vi "Emballage_BDD_correspondance_Code_barre.vi"(7 "tableau des codes barres":string[](array[string]), 8 "entrée d'erreur (pas d'erreur)":errorcluster, 9 "tableau des produits code FAS":string[](array[string]), 10 "Etiquette scanné":string, 11 "MulticolumnListbox en entrée":refnum<vi>) -> (0 "sortie d'erreur":errorcluster, 1 "index_produit":i32, 2 "message":string, 3 "Produit Code FAS":string)   [LabVIEW 2020]
uses:
  Modules/FS/60_FS_Controles/60_FS_SetGet.ctl
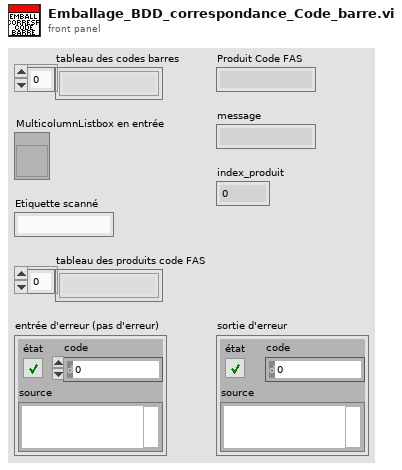
[diagram p1: front panel]
types:
  T1 = typedef "60_FS_SetGet.ctl" = enum16{"set", "get"}
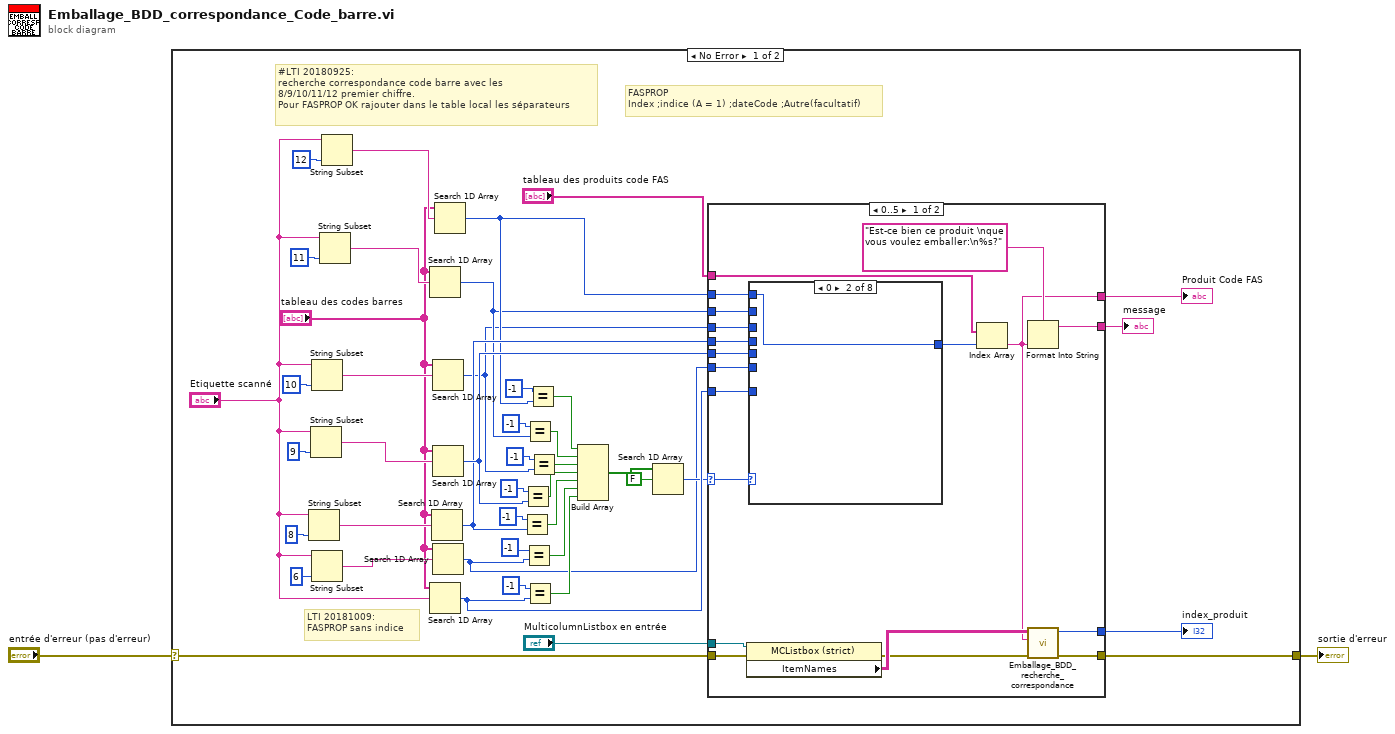
[diagram p0: block diagram]
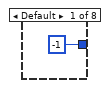
[diagram p2: hidden frame]
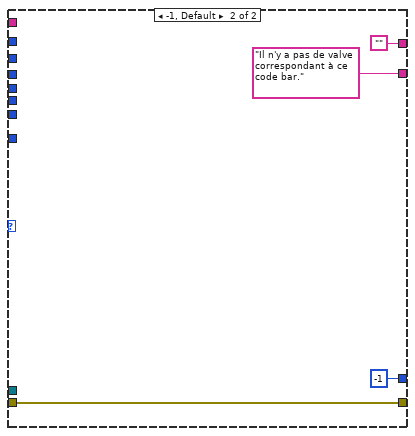
[diagram p9: hidden frame]
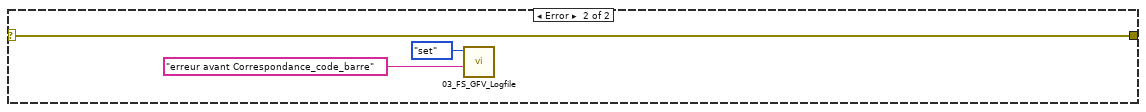
[diagram p10: hidden frame]
diagram:
  n1 = case shown="No Error" "entrée d'erreur (pas d'erreur)" {
    selector: "entrée d'erreur (pas d'erreur)" -> [w18 w81]
    tunnel: [w17 w81] -> w1
    frame No Error {
      # "LTI 20181009:\nFASPROP sans indice"
      # "#LTI 20180925:\nrecherche correspondance code barre avec les \n8/9/10/11/12 premier chiffre.\nPour FASPROP OK rajouter dans le table local les séparateurs"
      # "FASPROP\nIndex ;indice (A = 1) ;dateCode ;Autre(facultatif)"
      n2 = String Subset(string="Etiquette scanné", length (rest)=8 ("longueur (reste)")) -> (substring=w23:string)  [unwired: 1 in]
      n3 = String Subset(string="Etiquette scanné", length (rest)=9 ("longueur (reste)")) -> (substring=w41:string)  [unwired: 1 in]
      n4 = String Subset(string="Etiquette scanné", length (rest)=10 ("longueur (reste)")) -> (substring=w31:string)  [unwired: 1 in]
      n5 = String Subset(string="Etiquette scanné", length (rest)=6 ("longueur (reste)")) -> (substring=w8:string)  [unwired: 1 in]
      n6 = String Subset(string="Etiquette scanné", length (rest)=11 ("longueur (reste)")) -> (substring=w30:string)  [unwired: 1 in]
      n7 = String Subset(string="Etiquette scanné", length (rest)=12 ("longueur (reste)")) -> (substring=w28:string)  [unwired: 1 in]
      n8 = Search 1D Array(1D array="tableau des codes barres", element=w30) -> (index of element=w37:i32)  [unwired: 1 in]
      n9 = Search 1D Array(1D array="tableau des codes barres", element="Etiquette scanné") -> (index of element=w47:i32)  [unwired: 1 in]
      n10 = Search 1D Array(1D array="tableau des codes barres", element=w23) -> (index of element=w39:i32)  [unwired: 1 in]
      n11 = Search 1D Array(1D array="tableau des codes barres", element=w31) -> (index of element=w36:i32)  [unwired: 1 in]
      n12 = Search 1D Array(1D array="tableau des codes barres", element=w41) -> (index of element=w43:i32)  [unwired: 1 in]
      n13 = Search 1D Array(1D array="tableau des codes barres", element=w8) -> (index of element=w4:i32)  [unwired: 1 in]
      n14 = Search 1D Array(1D array="tableau des codes barres", element=w28) -> (index of element=w38:i32)  [unwired: 1 in]
      n15 = Equal?(x=-1, y=w39) -> (x = y?=w12:bool)
      n16 = Equal?(x=-1, y=w43) -> (x = y?=w13:bool)
      n17 = Equal?(x=-1, y=w4) -> (x = y?=w5:bool)
      n18 = Equal?(x=-1, y=w37) -> (x = y?=w15:bool)
      n19 = Equal?(x=-1, y=w47) -> (x = y?=w6:bool)
      n20 = Equal?(x=-1, y=w38) -> (x = y?=w16:bool)
      n21 = Equal?(x=-1, y=w36) -> (x = y?=w14:bool)
      n22 = Build Array(w16, w15, w14, w13, w12, w5, w6) -> (w26:bool[])
      n23 = Search 1D Array(1D array=w26, element=FALSE ("élément")) -> (index of element=w35:i32)  [unwired: 1 in]
      n24 = case shown="0..5" w35 {
        selector: w35 -> [w58 _]
        tunnel: "tableau des produits code FAS" -> [w66 _]
        tunnel: [w64 "Il n'y a pas de valve correspondant à ce code bar."] -> w21
        tunnel: [w61 ""] -> w45
        tunnel: w18 -> [w63 w76]
        tunnel: [w49 w76] -> w17
        tunnel: w36 -> [w56 _]
        tunnel: w37 -> [w55 _]
        tunnel: w38 -> [w54 _]
        tunnel: w39 -> [w53 _]
        tunnel: w43 -> [w52 _]
        tunnel: [w60 -1 ("élément")] -> w44
        tunnel: w47 -> [w51 _]
        tunnel: "MulticolumnListbox en entrée" -> [w59 _]
        tunnel: w4 -> [w48 _]
        frame 0..5 {
          n25 = property on="Nœud de propriété" class="MCListbox (strict)"(reference=w59, error in=w63) -> (error out=w50:errorcluster, "ItemNames"=w62:string[][])  [unwired: 1 out]
          n26 = case shown="0" w58 {
            tunnel: [-1 ("index of element") w68 w69 w70 w71 w72 w73 w74] -> w57
            tunnel: w56 -> [_ _ _ w70 _ _ _ _]
            tunnel: w55 -> [_ _ w69 _ _ _ _ _]
            tunnel: w54 -> [_ w68 _ _ _ _ _ _]
            tunnel: w53 -> [_ _ _ _ _ w72 _ _]
            tunnel: w52 -> [_ _ _ _ w71 _ _ _]
            tunnel: w51 -> [_ _ _ _ _ _ _ w74]
            tunnel: w48 -> [_ _ _ _ _ _ w73 _]
            frame Default {
            }
            frame 0 {
            }
            frame 1 {
            }
            frame 2 {
            }
            frame 3 {
            }
            frame 4 {
            }
            frame 5 {
            }
            frame 6 {
            }
          }
          n27 = Index Array(array=w66, index=w57) -> (element=w61:string)
          n28 = Format Into String(format string="Est-ce bien ce produit \nque vous voulez emballer:\n%s?", w61) -> (resulting string=w64:string)  [unwired: 2 in, 1 out]
          n29 = call "Emballage_BDD_recherche_correspondance.vi"("Error in"=w50, "Chaîne"=w61, "Tableau_IN"=w62) -> ("Error out"=w49:errorcluster, "élément"=w60:i32)  [unwired: 6 in, 1 out]
        }
        frame -1, Default {
        }
      }
      "Produit Code FAS" <- w45
      "index_produit" <- w44
      "message" <- w21
    }
    frame Error {
      n30 = call "03_FS_GFV_Logfile.vi"("Chaîne"="erreur avant Correspondance_code_barre", "States"=60_FS_SetGet."set") -> ()  [unwired: 8 in, 2 out]
    }
  }
  "sortie d'erreur" <- w1
